vi "Get Bitfiles Path.vi"() -> (0 "Bitfiles path":path)   [LabVIEW 2018, in "FPGA Addon Load And Parse Bitfile Unit Tests.lvclass"]
uses:
  FPGA Addon Load And Parse Bitfile Unit Tests.lvclass
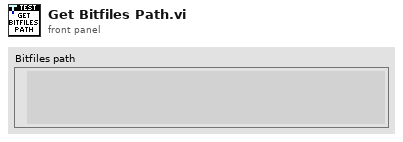
[diagram p1: front panel]
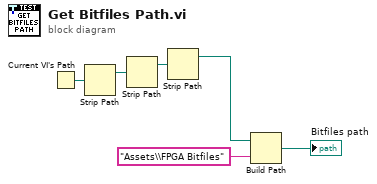
[diagram p0: block diagram]
diagram:
  n1 = Current VI's Path() -> (path=w1:path)
  n2 = Strip Path(path=w1) -> (stripped path=w2:path)  [unwired: 1 out]
  n3 = Strip Path(path=w2) -> (stripped path=w3:path)  [unwired: 1 out]
  n4 = Strip Path(path=w3) -> (stripped path=w4:path)  [unwired: 1 out]
  n5 = Build Path(base path=w4, name or relative path="Assets\\FPGA Bitfiles") -> (appended path=→"Bitfiles path":path)
